vi "Lat-Long M-S to Deg.vi"(9 "Long Min-Sec":string="12214.0164,W", 11 "Lat Min-Sec":string="4728.3818,N") -> (0 "Long Deg String":string, 1 "Long Deg":dbl, 2 "lat Deg String":string, 3 "Lat Deg":dbl)   [LabVIEW 2024, in "EQMF.lvlib" / "Math Utils.lvlib"]
uses:
  Math Utils.lvlib
  <vilib>/Utility/error.llb/Trim Whitespace One-Sided.vi
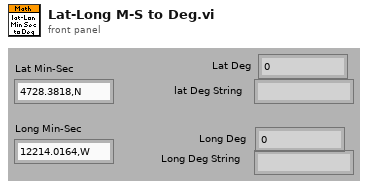
[diagram p1: front panel]
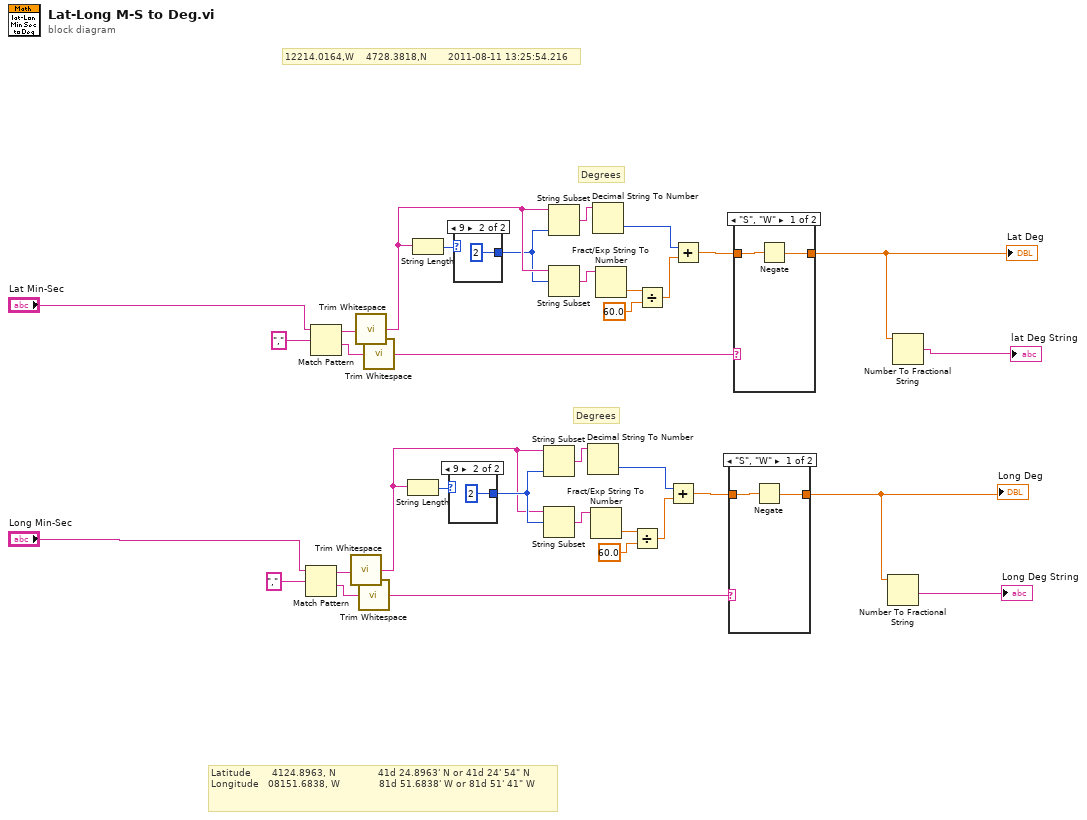
[diagram p0: block diagram]
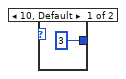
[diagram p2: hidden frame]
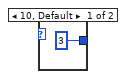
[diagram p4: hidden frame]
diagram:
  # "Degrees"
  # "12214.0164,W    4728.3818,N       2011-08-11 13:25:54.216"
  # "Degrees"
  # "Latitude       4124.8963, N              41d 24.8963' N or 41d 24' 54\" N \nLongitude   08151.6838, W             81d 51.6838' W or 81d 51' 41\" W"
  n1 = Match Pattern(string="Long Min-Sec", regular expression=",") -> (before substring=w11:string, after substring=w2:string)  [unwired: 1 in, 2 out]
  n2 = Match Pattern(string="Lat Min-Sec", regular expression=",") -> (before substring=w18:string, after substring=w27:string)  [unwired: 1 in, 2 out]
  n3 = call <vilib>:"Trim Whitespace.vi"("string"=w11) -> ("trimmed string"=w12:string)  [unwired: 1 in]
  n4 = call <vilib>:"Trim Whitespace.vi"("string"=w18) -> ("trimmed string"=w17:string)  [unwired: 1 in]
  n5 = call <vilib>:"Trim Whitespace.vi"("string"=w2) -> ("trimmed string"=w10:string)  [unwired: 1 in]
  n6 = call <vilib>:"Trim Whitespace.vi"("string"=w27) -> ("trimmed string"=w19:string)  [unwired: 1 in]
  n7 = String Length(string=w12) -> (length=w14:i32)
  n8 = String Length(string=w17) -> (length=w15:i32)
  n9 = case shown="9" w14 {
    tunnel: [3 2] -> w13
    frame 10, Default {
    }
    frame 9 {
    }
  }
  n10 = case shown="9" w15 {
    tunnel: [3 2] -> w16
    frame 10, Default {
    }
    frame 9 {
    }
  }
  n11 = String Subset(string=w12, length (rest)=w13) -> (substring=w3:string)  [unwired: 1 in]
  n12 = String Subset(string=w12, offset (0)=w13) -> (substring=w4:string)  [unwired: 1 in]
  n13 = String Subset(string=w17, length (rest)=w16) -> (substring=w26:string)  [unwired: 1 in]
  n14 = String Subset(string=w17, offset (0)=w16) -> (substring=w25:string)  [unwired: 1 in]
  n15 = Decimal String To Number(string=w3) -> (number=w7:i32)  [unwired: 2 in, 1 out]
  n16 = Fract/Exp String To Number(string=w4) -> (number=w5:dbl)  [unwired: 3 in, 1 out]
  n17 = Decimal String To Number(string=w26) -> (number=w22:i32)  [unwired: 2 in, 1 out]
  n18 = Fract/Exp String To Number(string=w25) -> (number=w24:dbl)  [unwired: 3 in, 1 out]
  n19 = Divide(x=w5, y=60.0) -> (x/y=w8:dbl)
  n20 = Divide(x=w24, y=60.0) -> (x/y=w21:dbl)
  n21 = Add(x=w7, y=w8) -> (x+y=w9:dbl)
  n22 = Add(x=w22, y=w21) -> (x+y=w20:dbl)
  n23 = case shown="\"S\", \"W\"" w10 {
    tunnel: w9 -> [w40 w41]
    tunnel: [w39 w41] -> w30
    frame "S", "W" {
      n24 = Negate(x=w40) -> (-x=w39:dbl)
    }
    frame "E", "N", Default {
    }
  }
  "Long Deg" <- w30
  n25 = case shown="\"S\", \"W\"" w19 {
    tunnel: w20 -> [w43 w44]
    tunnel: [w42 w44] -> w33
    frame "S", "W" {
      n26 = Negate(x=w43) -> (-x=w42:dbl)
    }
    frame "E", "N", Default {
    }
  }
  "Lat Deg" <- w33
  n27 = Number To Fractional String(number=w30) -> (F-format string=→"Long Deg String":string)  [unwired: 3 in]
  n28 = Number To Fractional String(number=w33) -> (F-format string=→"lat Deg String":string)  [unwired: 3 in]
